vi "add to buffer.vi"(10 "read data":string, 11 "buffer in":T1[](array[typedef])) -> (3 "buffer out":T1[](array[typedef]))   [LabVIEW 2012, in "RTU Data Unit.lvclass"]
uses:
  RTU Data Unit.lvclass
  buffer element.ctl
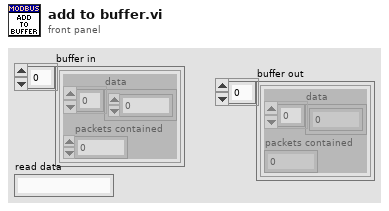
[diagram p1: front panel]
types:
  T1 = typedef "RTU Data Unit.lvclass/buffer element.ctl" = cluster{"data":u8[], "packets contained":i32}
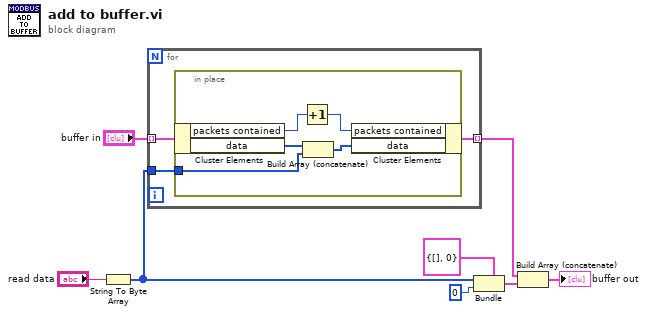
[diagram p0: block diagram]
diagram:
  n1 = String To Byte Array(string="read data") -> (unsigned byte array=w3:u8[])
  n2 = for {
    tunnel: "buffer in" -> [w11] mode=indexing
    tunnel: [w10] -> w4 mode=indexing
    tunnel: w3 -> [w9]
    n3 = in-place {
      in-place-border: w9 -> [w14]
      n4 = in-place-cluster #1(w11) -> ("packets contained"=w13:i32, "data"=w16:u8[])
      n5 = Increment(x=w13) -> (x+1=w12:i32)
      n6 = Build Array (concatenate)(w16, w14) -> (w15:u8[])
      n7 = in-place-cluster #1("packets contained"=w12, "data"=w15) -> (w10:T1)
    }
  }
  n8 = Bundle(cluster=T1 {"data"=[], "packets contained"=0}, "data"=w3, "packets contained"=0) -> (w6:T1)
  n9 = Build Array (concatenate)(w4, w6) -> (→"buffer out":T1[])
